vi "Configure Library in Memory for Build.vi"(7 "target name (My Computer)":string="My Computer", 9 "enable debugging? (F)":bool, 10 "save VIs? (T)":bool=TRUE, 11 "library name":string="DSF Core.lvlib") -> (0 "error out":errorcluster)   [LabVIEW 2020, in "Build Automation.lvlib"]
uses:
  Build Automation.lvlib
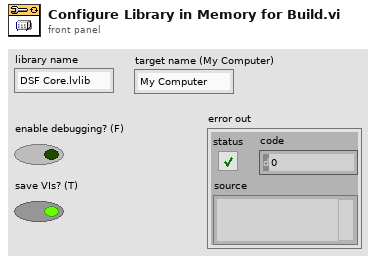
[diagram p1: front panel]
types:
  T1 = enum16{"Share clones between instances", "Preallocate clone for each instance"}
  T2 = cluster{"Status Message":refnum<data-value>, "Progress":refnum<data-value>, "Stop":refnum<data-value>}
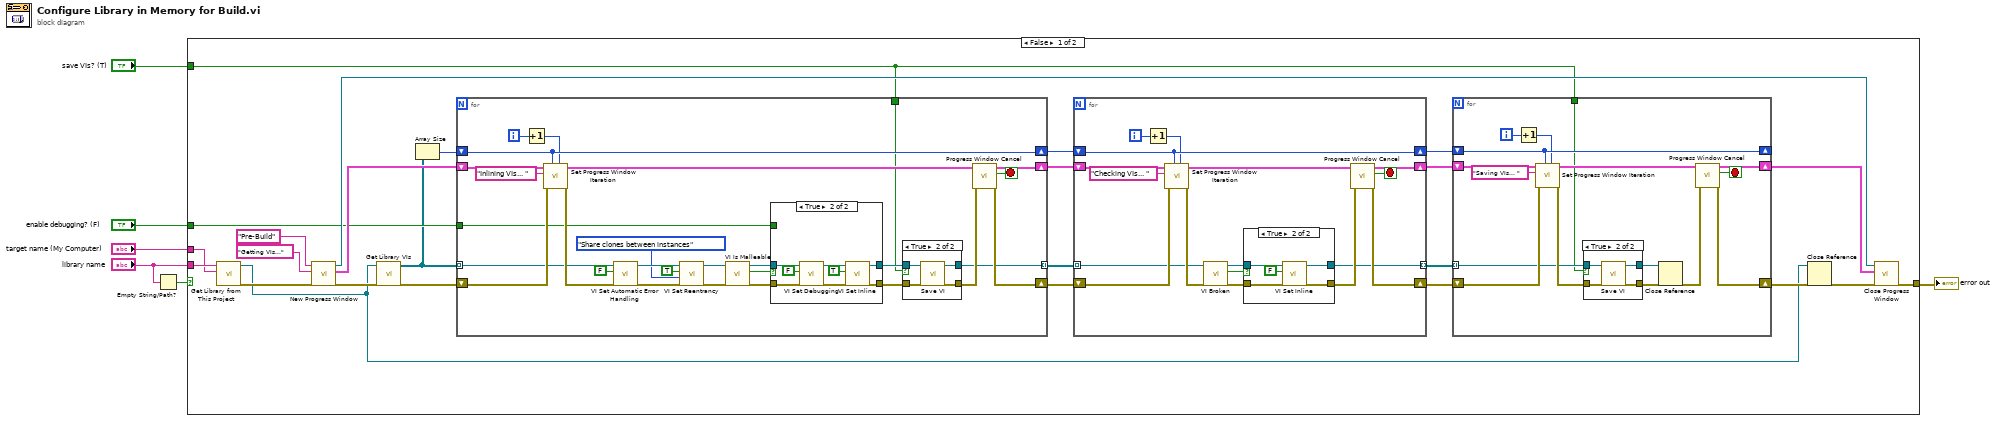
[diagram p0: block diagram]
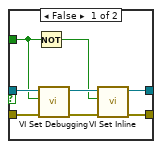
[diagram p3: hidden frame]
diagram:
  n1 = Empty String/Path?(string/path="library name") -> (empty?=w3:bool)
  n2 = case shown="False" w3 {
    tunnel: [w28 _] -> w6
    tunnel: "enable debugging? (F)" -> [w27 _]
    tunnel: "library name" -> [w10 _]
    tunnel: "save VIs? (T)" -> [w8 _]
    tunnel: "target name (My Computer)" -> [w9 _]
    frame False {
      n3 = call "Get Library from This Project.vi"("Target Name (My Computer)"=w9, "Library Name"=w10) -> ("error out"=w12:errorcluster, "Library Refnum"=w11:refnum<vi>)  [unwired: 8 in]
      n4 = call "New Progress Window.vi"("error in (no error)"=w12, "Initial Message"="Getting VIs...", "Window Title"="Pre-Build" ("WindowTitle")) -> ("error out"=w30:errorcluster, "DVRs"=w29:T2, "VI refnum"=w31:refnum<vi>)  [unwired: 6 in]
      n5 = call "Get Library VIs.vi"("error in (no error)"=w30, "library ref"=w11) -> ("error out"=w32:errorcluster, "vi refs"=w25:refnum<vi>[])  [unwired: 8 in]
      n6 = Array Size(array=w25) -> (size(s)=w26:i32)
      n7 = for {
        tunnel: w25 -> [w44] mode=indexing
        shift-right: [w58] -> w23
        shift-left: w29 -> [w49]
        shift-right: [w45] -> w21
        shift-left: w32 -> [w47]
        tunnel: w27 -> [w43]
        tunnel: [w35] -> w22 mode=indexing
        shift-right: [w42] -> w24
        shift-left: w26 -> [w42]
        tunnel: w8 -> [w36]
        i -> [w60]
        stop <- w59 stop-if-true
        n8 = Increment(x=w60) -> (x+1=w41:i32)
        n9 = call "Set Progress Window Iteration.vi"("current iteration"=w41, "total iterations"=w42, "error in (no error)"=w47, "Status Message"="Inlining VIs... ", "DVRs in"=w49) -> ("error out"=w46:errorcluster, "DVRs out"=w48:T2)  [unwired: 5 in]
        n10 = call "VI Set Automatic Error Handling.vi"("error in (no error)"=w46, "Automatic Error Handling"=FALSE, "vi ref in"=w44) -> ("error out"=w55:errorcluster, "vi ref out"=w56:refnum<vi>)  [unwired: 7 in]
        n11 = call "VI Set Reentrancy.vi"("error in (no error)"=w55, "Reentrancy Type (shared clone)"=T1."Share clones between instances" ("Reentrancy Type"), "Is Reentrant"=TRUE, "vi ref in"=w56) -> ("error out"=w53:errorcluster, "vi ref out"=w54:refnum<vi>)  [unwired: 6 in]
        n12 = call "VI Is Malleable.vi"("error in (no error)"=w53, "vi ref in"=w54) -> ("error out"=w52:errorcluster, "malleable VI?"=w50:bool, "vi ref out"=w51:refnum<vi>)  [unwired: 7 in]
        n13 = case shown="True" w50 {
          tunnel: [w72 w80] -> w38
          tunnel: [w71 w79] -> w39
          tunnel: w52 -> [w68 w77]
          tunnel: w51 -> [w69 w78]
          tunnel: w43 -> [w67 _]
          frame False {
            n14 = Not(x=w67) -> (.not. x?=w70:bool)
            n15 = call "VI Set Debugging.vi"("error in (no error)"=w68, "Allow Debugging"=w67, "vi ref in"=w69) -> ("error out"=w73:errorcluster, "vi ref out"=w74:refnum<vi>)  [unwired: 7 in]
            n16 = call "VI Set Inline.vi"("error in (no error)"=w73, "Inline VI"=w70, "vi ref in"=w74) -> ("error out"=w71:errorcluster, "vi ref out"=w72:refnum<vi>)  [unwired: 7 in]
          }
          frame True {
            n17 = call "VI Set Debugging.vi"("error in (no error)"=w77, "Allow Debugging"=FALSE, "vi ref in"=w78) -> ("error out"=w81:errorcluster, "vi ref out"=w82:refnum<vi>)  [unwired: 7 in]
            n18 = call "VI Set Inline.vi"("error in (no error)"=w81, "Inline VI"=TRUE, "vi ref in"=w82) -> ("error out"=w79:errorcluster, "vi ref out"=w80:refnum<vi>)  [unwired: 7 in]
          }
        }
        n19 = case shown="True" w36 {
          tunnel: w39 -> [w61 w66]
          tunnel: [w62 w65] -> w35
          tunnel: [w61 w64] -> w37
          tunnel: w38 -> [w62 w63]
          frame False {
          }
          frame True {
            n20 = call "Save VI.vi"("error in (no error)"=w66, "vi ref in"=w63) -> ("error out"=w64:errorcluster, "vi ref out"=w65:refnum<vi>)  [unwired: 8 in]
          }
        }
        n21 = call "Progress Window Cancel.vi"("error in (no error)"=w37, "DVRs in"=w48) -> ("error out"=w45:errorcluster, "cancelled"=w59:bool, "DVRs out"=w58:T2)  [unwired: 7 in]
      }
      n22 = for {
        tunnel: w22 -> [w88] mode=indexing
        shift-right: [w97] -> w20
        shift-left: w23 -> [w96]
        shift-right: [w93] -> w18
        shift-left: w21 -> [w94]
        shift-right: [w92] -> w19
        shift-left: w24 -> [w92]
        tunnel: [w83] -> w17 mode=indexing
        i -> [w99]
        stop <- w98 stop-if-true
        n23 = Increment(x=w99) -> (x+1=w91:i32)
        n24 = call "Set Progress Window Iteration.vi"("current iteration"=w91, "total iterations"=w92, "error in (no error)"=w94, "Status Message"="Checking VIs... ", "DVRs in"=w96) -> ("error out"=w89:errorcluster, "DVRs out"=w95:T2)  [unwired: 5 in]
        n25 = call "VI Broken.vi"("error in (no error)"=w89, "vi ref in"=w88) -> ("error out"=w86:errorcluster, "broken?"=w85:bool, "vi ref out"=w87:refnum<vi>)  [unwired: 7 in]
        n26 = case shown="True" w85 {
          tunnel: [w101 w106] -> w83
          tunnel: [w100 w105] -> w84
          tunnel: w86 -> [w100 w104]
          tunnel: w87 -> [w101 w102]
          frame False {
          }
          frame True {
            n27 = call "VI Set Inline.vi"("error in (no error)"=w104, "Inline VI"=FALSE, "vi ref in"=w102) -> ("error out"=w105:errorcluster, "vi ref out"=w106:refnum<vi>)  [unwired: 7 in]
          }
        }
        n28 = call "Progress Window Cancel.vi"("error in (no error)"=w84, "DVRs in"=w95) -> ("error out"=w93:errorcluster, "cancelled"=w98:bool, "DVRs out"=w97:T2)  [unwired: 7 in]
      }
      n29 = for {
        tunnel: w17 -> [w108] mode=indexing
        shift-right: [w120] -> w16
        shift-left: w20 -> [w119]
        shift-right: [w116] -> w14
        shift-left: w18 -> [w117]
        shift-right: [w115] -> _
        shift-left: w19 -> [w115]
        tunnel: w8 -> [w107]
        i -> [w122]
        stop <- w121 stop-if-true
        n30 = Increment(x=w122) -> (x+1=w114:i32)
        n31 = call "Set Progress Window Iteration.vi"("current iteration"=w114, "total iterations"=w115, "error in (no error)"=w117, "Status Message"="Saving VIs... ", "DVRs in"=w119) -> ("error out"=w109:errorcluster, "DVRs out"=w118:T2)  [unwired: 5 in]
        n32 = case shown="True" w107 {
          tunnel: w109 -> [w123 w128]
          tunnel: [w124 w127] -> w112
          tunnel: [w123 w126] -> w111
          tunnel: w108 -> [w124 w125]
          frame False {
          }
          frame True {
            n33 = call "Save VI.vi"("error in (no error)"=w128, "vi ref in"=w125) -> ("error out"=w126:errorcluster, "vi ref out"=w127:refnum<vi>)  [unwired: 8 in]
          }
        }
        n34 = Close Reference(reference=w112, error in (no error)=w111) -> (error out=w110:errorcluster)
        n35 = call "Progress Window Cancel.vi"("error in (no error)"=w110, "DVRs in"=w118) -> ("error out"=w116:errorcluster, "cancelled"=w121:bool, "DVRs out"=w120:T2)  [unwired: 7 in]
      }
      n36 = Close Reference(reference=w11, error in (no error)=w14) -> (error out=w13:errorcluster)
      n37 = call "Close Progress Window.vi"("error in (no error)"=w13, "DVRs in"=w16, "VI refnum"=w31) -> ("error out"=w28:errorcluster)  [unwired: 8 in]
    }
    frame True {
    }
  }
  "error out" <- w6
